vi "LWXPS_FirmwareVersionGet.vi"(0 "XPS Reference IN":refnum<k24>, 11 "LabVIEW error IN":errorcluster) -> (4 "XPS Reference OUT":refnum<k24>, 6 "Returned error code":i32, 8 "XPS Controller Version":string, 10 "XPS Error String":string, 15 "LabVIEW error OUT":errorcluster)   [LabVIEW 2014]
uses:
  D:/XPSQ8_LabView_Library/Development/Source/Dll/Newport.XPS.CommandInterface.dll
  Dll/Newport.XPS.CommandInterface.dll
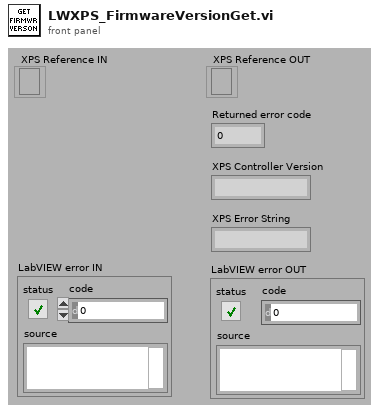
[diagram p1: front panel]
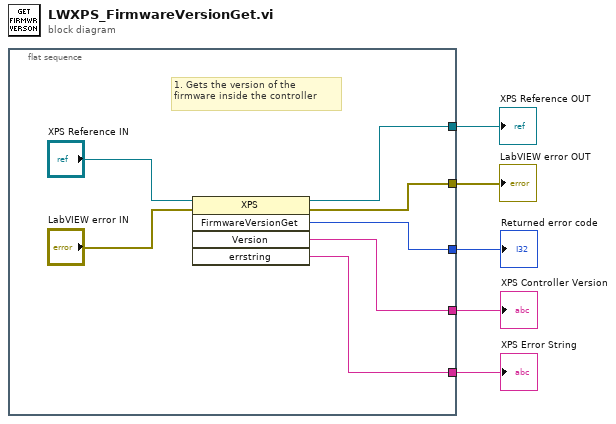
[diagram p0: block diagram]
diagram:
  n1 = flat-sequence {
    tunnel: [w11] -> w5
    tunnel: [w10] -> w4
    tunnel: [w9] -> w3
    tunnel: [w8] -> w2
    tunnel: [w7] -> w1
    frame #0 {
      # "1. Gets the version of the firmware inside the controller"
      n2 = invoke class="XPS" method="FirmwareVersionGet"(reference="XPS Reference IN", error in="LabVIEW error IN") -> (reference out=w9:refnum<k24>, error out=w8:errorcluster, "FirmwareVersionGet"=w7:i32, "Version"=w11:string, "errstring"=w10:string)  [unwired: 3 in]
    }
  }
  "XPS Controller Version" <- w5
  "XPS Error String" <- w4
  "XPS Reference OUT" <- w3
  "LabVIEW error OUT" <- w2
  "Returned error code" <- w1
